vi "HeartBeatDetectOffline1Simple.vi"() -> ()   [LabVIEW 2014, in "Phonocardiography.lvlib"]
uses:
  Phonocardiography.lvlib
  <vilib>/Waveform/WDTOps.llb/WDT Index Channel DBL.vi
  <vilib>/Waveform/WDTOps.llb/WDT Get Waveform Time Array DBL.vi
  <vilib>/Analysis/NI_AAL_SigProc.lvlib
panel:
  out "Peaks":cluster{dbl[], "Amplitudes":dbl[]}[](graph)=[{array[122880 elements], "Amplitudes"=array[122880 elements]}, {[0.2683937704472721, 1.0181964328893598, 1.7377038104855096, 2.4855473692602947, 3.2774489982847803, 4.117602629900593, 5.0497054685009335, 5.994733213940523, 6.895302722768209, 7.797557321695085, 8.691660475532698, 9.53679206192987, 10.39302687835089], "Amplitudes"=[0.31315447076575686, 0.3206463592501255, 0.30828679771720463, 0.3046863092516966, 0.3208257168568248, 0.33907754062759177, 0.3184735631174685, 0.2664009802503432, 0.3439713540857765, 0.30399089060543044, 0.30335101069011816, 0.3364507699677884, 0.30464834692469883]}]
  in  "Threshold mult":dbl=0.65 min=-1.0 max=1.0 step=0.05
  in  "width (threshold)":i32=30
  in  "File Path":path=path "C:/Users/Tamas/Documents/Projektek/Magzati szívhang/Nem babás/szep/nagy1.wav"
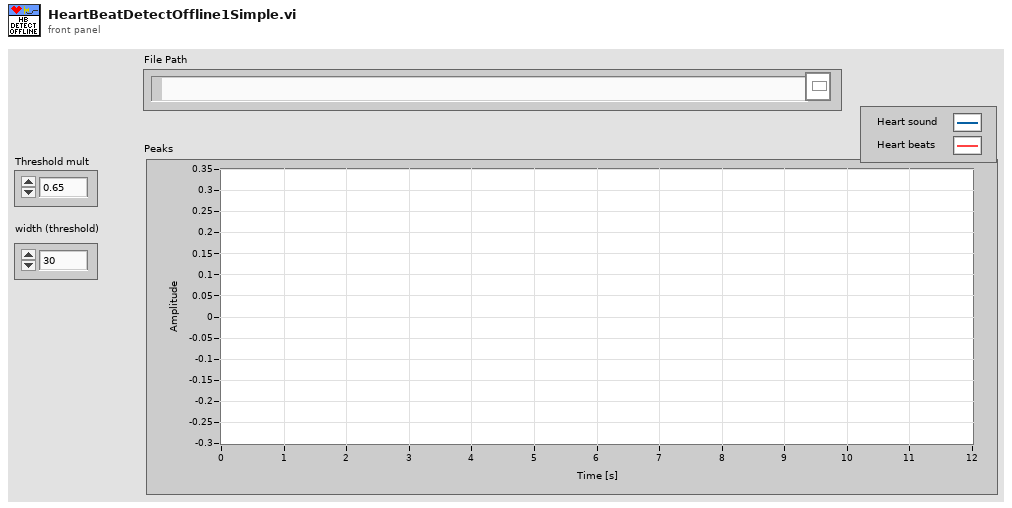
[diagram p1: front panel]
types:
  T1 = typedef "LVCursorListTypeDef.ctl" = cluster{"Name":string, "Color":u32, "Style":u8, "Point Style":u8, "Name Visible":bool, "Allow Drag":bool, "Cursor Mode":u32, "Plot":i32, "Index":i32, "Position":cluster{"X":dbl, "Y":dbl}, "X Scale":u32, "Y Scale":u32, "Watch Plots":i32[], "Watch All Plots":bool, "Plot Area":i32, "Label Offset":cluster{"X":dbl, "Y":dbl}}[]
  T2 = cluster{"Name":string, "Color":u32, "Style":u8, "Point Style":u8, "Name Visible":bool, "Allow Drag":bool, "Cursor Mode":u32, "Plot":i32, "Index":i32, "Position":cluster{"X":dbl, "Y":dbl}, "X Scale":u32, "Y Scale":u32, "Watch Plots":i32[], "Watch All Plots":bool, "Plot Area":i32, "Label Offset":cluster{"X":dbl, "Y":dbl}}
  T3 = cluster{"Name":string, "Color":u32, "Style":u8, "Point Style":u8, "Name Visible":bool, "Allow Drag":bool, "Cursor Mode":u32, "Plot":i32, "Index":i32, "Position":cluster{"X":dbl, "Y":dbl}, "X Scale":u32, "Y Scale":u32, "Watch Plots":i32[], "Watch All Plots":bool, "Plot Area":i32, "Label Offset":cluster{"X":dbl, "Y":dbl}}[]
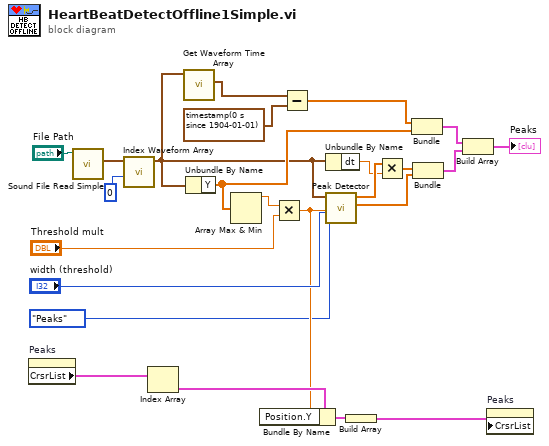
[diagram p0: block diagram]
diagram:
  n1 = property on="Peaks" class="XYGraph (strict)"() -> ("CrsrList"=w10:T1)  [unwired: 2 in, 2 out]
  n2 = call <vilib>:"Sound File Read Simple.vi"("path"="File Path") -> ("data"=w23:waveform(dbl)[])  [unwired: 7 in, 3 out]
  n3 = call-poly <vilib>:"Index Waveform Array.vi"("index"=0, "waveform array"=w23) -> ("waveform"=w1:waveform(dbl))  [unwired: 8 in, 1 out]
  n4 = Index Array(array=w10) -> (element=w19:T2)  [unwired: 1 in]
  n5 = call-poly <vilib>:"Get Waveform Time Array.vi"("waveform in"=w1) -> ("X array"=w8:timestamp[])  [unwired: 9 in, 1 out]
  n6 = Unbundle By Name(w1) -> ("Y"=w5:dbl[])
  n7 = Array Max & Min(array=w5) -> (max value=w18:dbl)  [unwired: 3 out]
  n8 = Multiply(x=w18, y="Threshold mult") -> (x*y=w15:dbl)
  n9 = Bundle By Name(cluster=w19, "Position.Y"=w15) -> (w17:T2)
  n10 = Subtract(x=w8, y=timestamp(0 s since 1904-01-01) ("Xo")) -> (x-y=w6:dbl[])
  n11 = Unbundle By Name(w1) -> ("dt"=w13:dbl)
  n12 = call <vilib>:"Peak Detector.vi"("peaks/valleys"=enum32{"Peaks", "Valleys"}."Peaks", "width"="width (threshold)", "threshold"=w15, "X"=w1) -> ("Amplitudes"=w12:dbl[], "Locations"=w14:dbl[])  [unwired: 3 in, 3 out]
  n13 = Build Array(w17) -> (w9:T3)
  n14 = Multiply(x=w14, y=w13) -> (x*y=w2:dbl[])
  n15 = Bundle(w6, "Y"=w5) -> (w4:cluster{dbl[], "Y":dbl[]})  [unwired: 1 in]
  n16 = Bundle(w2, "Amplitudes"=w12) -> (w20:cluster{dbl[], "Amplitudes":dbl[]})  [unwired: 1 in]
  n17 = Build Array(w4, w20) -> (→"Peaks":cluster{dbl[], "Amplitudes":dbl[]}[])
  n18 = property on="Peaks" class="XYGraph (strict)"("CrsrList"=w9) -> ()  [unwired: 2 in, 2 out]
